vi "ArrayToExcel.vi"() -> ()   [LabVIEW 2020]
uses:
  <vilib>/Analysis/NI_AALBase.lvlib
panel:
  out "SEÑALES":dbl[][](graph)
  out "F-format string":string[][](array[string])
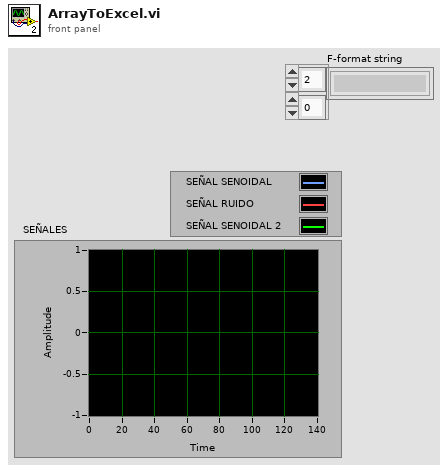
[diagram p1: front panel]
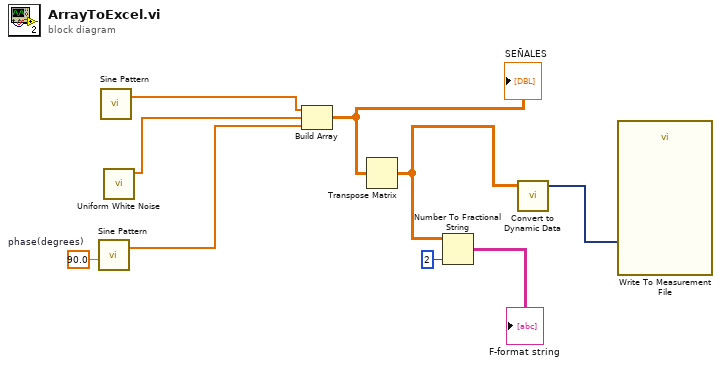
[diagram p0: block diagram]
diagram:
  w6 = 90.0  # phase(degrees)
  n1 = call <vilib>:"Sine Pattern.vi"("phase(degrees)"=w6) -> ("Sinusoidal Pattern"=w7:dbl[])  [unwired: 3 in, 1 out]
  n2 = call <vilib>:"Sine Pattern.vi"() -> ("Sinusoidal Pattern"=w9:dbl[])  [unwired: 4 in, 1 out]
  n3 = call <vilib>:"Uniform White Noise.vi"() -> ("uniform white noise"=w8:dbl[])  [unwired: 10 in, 1 out]
  n4 = Build Array "Build Array"(w9, w8, w7) -> (w3:dbl[][])
  "SEÑALES" <- w3
  n5 = Transpose Matrix(1:w3) -> (0:w2:dbl[][])
  n6 = Number To Fractional String(number=w2, precision (6)=i16 2) -> (F-format string=→"F-format string":string[][])  [unwired: 2 in]
  n7 = call "Convert to Dynamic Data"("2D Array"=w2) -> ("Dynamic Data Type"=w1:dynamicdata)  [unwired: 3 in]
  n8 = call "Write To Measurement File"("Signals"=w1) -> ()  [unwired: 16 in, 3 out]
